vi "Table Control Active Cell.vi"(6 "Cell Background Color":T2={"ColHeader"=14869218, "Normal"=16777226, "HighLight"=3381759}, 8 "error in (no error)":errorcluster, 9 "MousePoint":T1, 10 "Editable Columns":i32[](array[numeric]), 11 "Tbl Refnum":refnum<vi>) -> (0 "error out":errorcluster, 2 "RowInRange":bool, 3 "Tbl Refnum out":refnum<vi>)   [LabVIEW 2021]
uses:
  <vilib>/Utility/miscctls.llb/LVRowAndColumnTypeDef.ctl
  <vilib>/Utility/miscctls.llb/LVPositionTypeDef.ctl
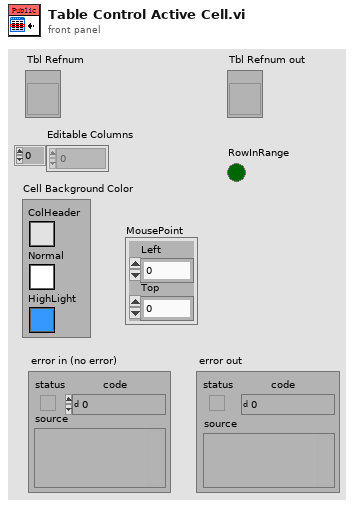
[diagram p1: front panel]
types:
  T1 = typedef "LVPositionTypeDef.ctl" = cluster{"Left":i32, "Top":i32}
  T2 = cluster{"ColHeader":u32, "Normal":u32, "HighLight":u32}
  T3 = typedef "LVRowAndColumnTypeDef.ctl" = cluster{"Row":i32, "Column":i32}
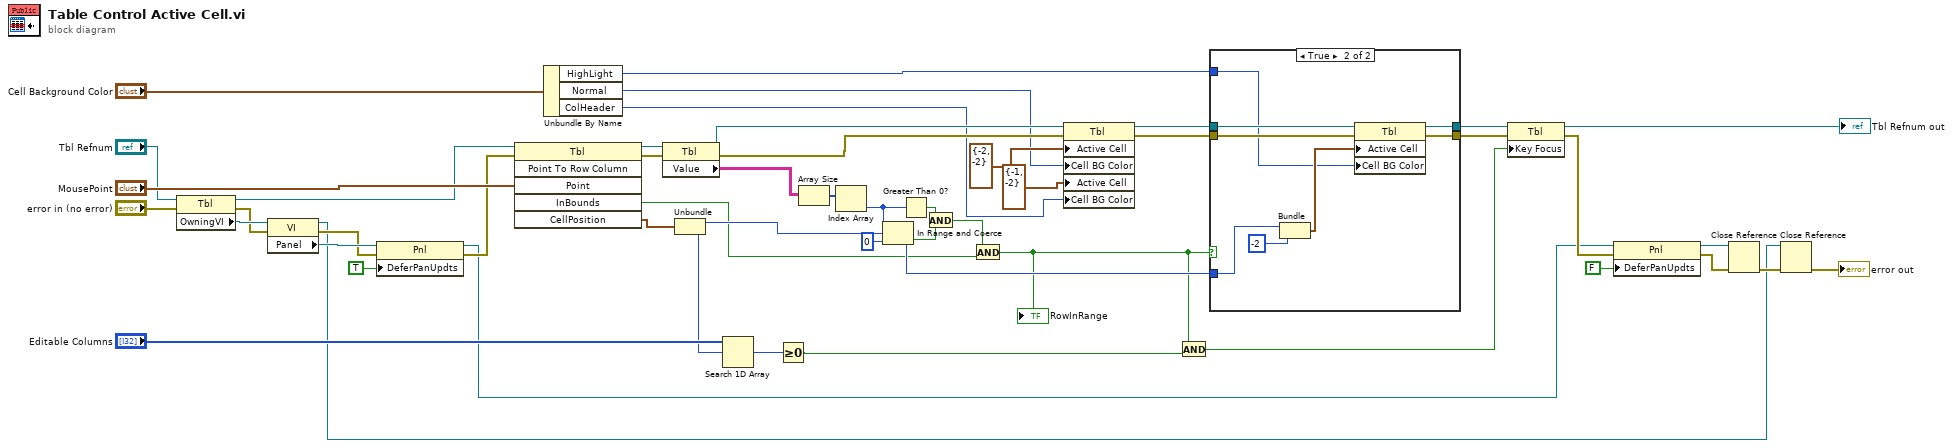
[diagram p0: block diagram]
diagram:
  n1 = property class="Tbl"(reference="Tbl Refnum", error in="error in (no error)") -> (reference out=w20:refnum<vi>, error out=w18:errorcluster, "OwningVI"=w19:refnum<vi>)
  n2 = property class="VI"(reference=w19, error in=w18) -> (reference out=w7:refnum<vi>, error out=w16:errorcluster, "Panel"=w17:refnum<vi>)
  n3 = property class="Pnl"(reference=w17, error in=w16, "DeferPanUpdts"=TRUE ("Defer Panel Updates")) -> (reference out=w12:refnum<vi>, error out=w15:errorcluster)
  n4 = invoke class="Tbl" method="Point To Row Column"(reference=w20, error in=w15, "Point"="MousePoint") -> (reference out=w50:refnum<vi>, error out=w41:errorcluster, "InBounds"=w2:bool, "CellPosition"=w49:T3)  [unwired: 3 in, 2 out]
  n5 = Unbundle By Name("Cell Background Color") -> ("HighLight"=w26:u32, "Normal"=w30:u32, "ColHeader"=w29:u32)
  n6 = property class="Tbl"(reference=w50, error in=w41) -> (reference out=w33:refnum<vi>, error out=w32:errorcluster, "Value"=w42:string[][])
  n7 = Unbundle(w49) -> ("Row"=w48:i32, "Column"=w37:i32)
  n8 = Search 1D Array(1D array="Editable Columns", element=w37) -> (index of element=w36:i32)  [unwired: 1 in]
  n9 = Greater Or Equal To 0?(x=w36) -> (x >= 0?=w5:bool)
  n10 = Array Size(array=w42) -> (size(s)=w46:i32[])
  n11 = Index Array(array=w46) -> (element=w45:i32)  [unwired: 1 in]
  n12 = In Range and Coerce(upper limit=w45, x=w48, lower limit=0) -> (coerced(x)=w39:i32, In Range?=w44:bool)
  n13 = Greater Than 0?(x=w45) -> (x > 0?=w43:bool)
  n14 = And(x=w43, y=w44) -> (x .and. y?=w3:bool)
  n15 = And(x=w3, y=w2) -> (x .and. y?=w1:bool)
  "RowInRange" <- w1
  n16 = property on="Property Node" class="Tbl"(reference=w33, error in=w32, "Active Cell"=T3 {"Row"=-2, "Column"=-2} ("Active Cell:Active Cell"), "Cell BG Color"=w30, "Active Cell"=T3 {"Row"=-1, "Column"=-2} ("Active Cell:Active Cell"), "Cell BG Color"=w29) -> (reference out=w28:refnum<vi>, error out=w27:errorcluster)
  n17 = And(x=w1, y=w5) -> (x .and. y?=w4:bool)
  n18 = case shown="True" w1 {
    tunnel: w39 -> [_ w60]
    tunnel: w28 -> [w52 w57]
    tunnel: w27 -> [w51 w56]
    tunnel: w26 -> [_ w55]
    tunnel: [w52 w54] -> w25
    tunnel: [w51 w53] -> w24
    frame False {
    }
    frame True {
      n19 = Bundle("lower limit"=w60, "Row"=-2) -> (w58:cluster{"lower limit":i32, "Row":i32})  [unwired: 1 in]
      n20 = property on="Property Node" class="Tbl"(reference=w57, error in=w56, "Active Cell"=w58, "Cell BG Color"=w55) -> (reference out=w54:refnum<vi>, error out=w53:errorcluster)
    }
  }
  n21 = property on="Property Node" class="Tbl"(reference=w25, error in=w24, "Key Focus"=w4) -> (reference out=→"Tbl Refnum out":refnum<vi>, error out=w13:errorcluster)
  n22 = property class="Pnl"(reference=w12, error in=w13, "DeferPanUpdts"=FALSE ("Defer Panel Updates")) -> (reference out=w10:refnum<vi>, error out=w9:errorcluster)
  n23 = Close Reference(reference=w10, error in (no error)=w9) -> (error out=w8:errorcluster)
  n24 = Close Reference(reference=w7, error in (no error)=w8) -> (error out=→"error out":errorcluster)
